vi "LIMITKdll.vi"(8 "error in (no error)":errorcluster, 11 "Inputs":T2) -> (0 "error out":errorcluster, 3 "Outputs":T1)   [LabVIEW 2021]
doc: "subroutine LIMITKdll(htyp, icomp, t, D, p, tmin, tmax, dmax, pmax, ierr, herr, htyp_length, herr_length)\n\nReturns limits of a property model (read in from the .fld files) for\na mixture component and/or checks input t, D, p against those limits\n\nThis routine functions in the same manner as LIMITX except that the\ncomposition x is replaced by the component number icomp.\n\nAttempting calculations below the minimum temperature and/or above\nthe maximum density will result in an error. These will often\ncorrespond to a physically unreasonable state; also many equations of\nstate do not extrapolate reliably to lower T's and higher D's.\n\nA warning is issued if the temperature is above the maximum but below\n1.5 times the maximum; similarly pressures up to twice the maximum\nresult in only a warning. Most equations of state may be\nextrapolated to higher T's and P's. Temperatures and/or pressures\noutside these extended limits will result in an error.\n\nN.B.--all inputs must be specified, if one or more are not\n available, (or not applicable as in case of surface tension)\n use reasonable values, such as:\n t = tnbp\n D = 0\n p = 0\n\nINPUTS:\nhtyp -- flag indicating which models are to be checked [character*3]\n 'EOS': equation of state for thermodynamic properties\n 'ETA': viscosity\n 'TCX': thermal conductivity\n 'STN': surface tension\nicomp -- component number in mixture; 1 for pure fluid\nt -- temperature [K]\nD -- molar density [mol/L]\np -- pressure [kPa]\n \nOUTPUTS:\ntmin -- minimum temperature for model specified by htyp [K]\ntmax -- maximum temperature [K]\ndmax -- maximum density [mol/L]\npmax -- maximum pressure [kPa]\nierr -- error flag: 0 = all inputs within limits otherwise one or more inputs outside limits:\n -1 = 1.5*tmax > t > tmax\n 1 = t < tmin or t > 1.5*tmax\n 2 = D > Dmax or D < 0\n -4 = 2*pmax > p > pmax\n 4 = p < 0 or p > 2*pmax\n 16 = p>pmelt\n -16 = t<ttrp (important for water)\n if multiple inputs are outside limits, ierr = abs[sum(ierr)]\n with the sign determined by the most severe excursion\n (ierr > 0 indicate an error--calculations not possible,\n ierr < 0 indicate a warning--results may be questionable)\nherr -- error string\nhtyp_length -- length of variable htyp (default: 3)\nherr_length -- length of variable herr (default: 255)"
uses:
  REFPROP.dll
panel:
  # "REFPROP-LIMITKdll.vi"
  # "void  LIMITKdll(CStr htyp, int32_t *icomp, double *t, double *D, double *p, double *tmin, double *tmax, double *dmax, double *pmax, int32_t *ierr, CStr herr, int32_t htyp_length, int32_t herr_length)"
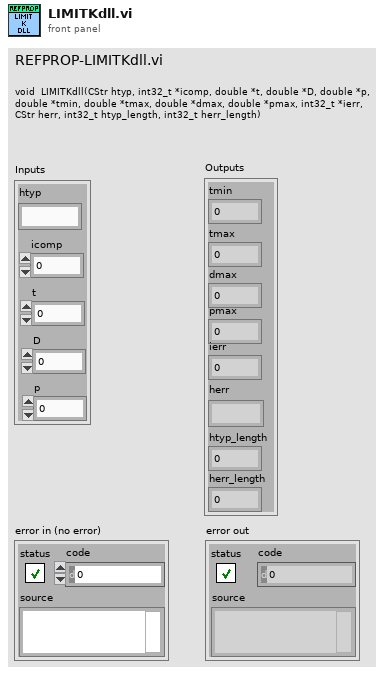
[diagram p1: front panel]
types:
  T1 = cluster{"tmin":dbl, "tmax":dbl, "dmax":dbl, "pmax":dbl, "ierr":i32, "herr":string, "htyp_length":i32, "herr_length":i32}
  T2 = cluster{"htyp":string, "icomp":i32, "t":dbl, "D":dbl, "p":dbl}
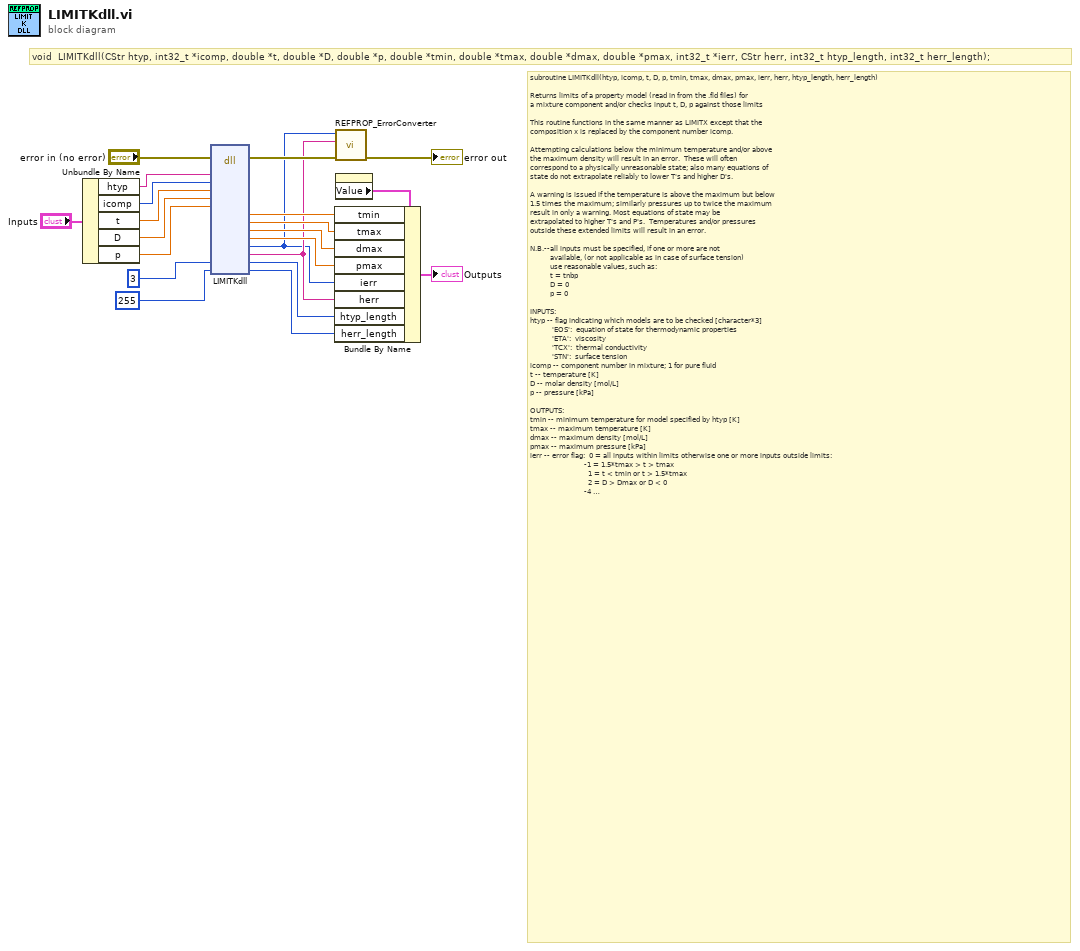
[diagram p0: block diagram]
diagram:
  # "void  LIMITKdll(CStr htyp, int32_t *icomp, double *t, double *D, double *p, double *tmin, double *tmax, double *dmax, double *pmax, int32_t *ierr, CStr herr, int32_t htyp_length, int32_t herr_length);"
  # "subroutine LIMITKdll(htyp, icomp, t, D, p, tmin, tmax, dmax, pmax, ierr, herr, htyp_length, herr_length)\n\nReturns limits of a property model (read in from the .fld files) for\na mixture component and/or checks input t, D, p against those limits\n\nThis routine functions in the same manner as LIMITX except that the\ncomposition x is replaced by the component number icomp.\n\nAttempting calculations below the minimum temperature and/or above\nthe maximum density will result in an error.  These will often\ncorrespond to a physically unreasonable state; also many equations of\nstate do not extrapolate reliably to lower T's and higher D's.\n\nA warning is issued if the temperature is above the maximum but below\n1.5 times the maximum; similarly pressures up to twice the maximum\nresult in only a warning. Most equations of state may be\nextrapolated to higher T's and P's.  Temperatures and/or pressures\noutside these extended limits will result in an error.\n\nN.B.--all inputs must be specified, if one or more are not\n          available, (or not applicable as in case of surface tension)\n          use reasonable values, such as:\n          t = tnbp\n          D = 0\n          p = 0\n\nINPUTS:\nhtyp -- flag indicating which models are to be checked [character*3]\n           'EOS':  equation of state for thermodynamic properties\n           'ETA':  viscosity\n           'TCX':  thermal conductivity\n           'STN':  surface tension\nicomp -- component number in mixture; 1 for pure fluid\nt -- temperature [K]\nD -- molar density [mol/L]\np -- pressure [kPa]\n   \nOUTPUTS:\ntmin -- minimum temperature for model specified by htyp [K]\ntmax -- maximum temperature [K]\ndmax -- maximum density [mol/L]\npmax -- maximum pressure [kPa]\nierr -- error flag:  0 = all inputs within limits otherwise one or more inputs outside limits:\n                           -1 = 1.5*tmax > t > tmax\n                             1 = t < tmin or t > 1.5*tmax\n                             2 = D > Dmax or D < 0\n                           -4 = 2*pmax > p > pmax\n                             4 = p < 0 or p > 2*pmax\n                           16 = p>pmelt\n                          -16 = t<ttrp (important for water)\n           if multiple inputs are outside limits, ierr = abs[sum(ierr)]\n           with the sign determined by the most severe excursion\n           (ierr > 0 indicate an error--calculations not possible,\n            ierr < 0 indicate a warning--results may be questionable)\nherr -- error string\nhtyp_length -- length of variable htyp (default: 3)\nherr_length -- length of variable herr (default: 255)"
  n1 = Unbundle By Name("Inputs") -> ("htyp"=w14:string, "icomp"=w13:i32, "t"=w12:dbl, "D"=w11:dbl, "p"=w15:dbl)
  n2 = dll-call lib="C:/Users/lauria/OneDrive - National Institute of Standards and Technology (NIST)/LabVIEW Projects/7 REFPROP/REFPROP-wrappers-master/REFPROP-wrappers-master/wrappers/Labview/REFPROP/REFPROP.*" fn="LIMITKdll"(error in="error in (no error)", "htyp"=w14, "icomp"=w13, "t"=w12, "D"=w11, "p"=w15, "htyp_length"=3 ("ln1"), "herr_length"=255 ("ln2")) -> (error out=w19:errorcluster, "tmin"=w8:dbl, "tmax"=w7:dbl, "dmax"=w6:dbl, "pmax"=w5:dbl, "ierr"=w1:i32, "herr"=w2:string, "htyp_length"=w4:i32, "herr_length"=w3:i32)  [unwired: 14 in, 1 out]
  n3 = call "REFPROP_ErrorConverter.vi"("error in (no error)"=w19, "Error Message"=w2, "Error Code"=w1) -> ("error out"=→"error out":errorcluster)  [unwired: 8 in]
  n4 = property on="Outputs" class="Clust (strict)"() -> ("Value"=w10:T1)  [unwired: 2 in, 2 out]
  n5 = Bundle By Name(cluster=w10, "tmin"=w8, "tmax"=w7, "dmax"=w6, "pmax"=w5, "ierr"=w1, "herr"=w2, "htyp_length"=w4, "herr_length"=w3) -> (→"Outputs":T1)
